vi "UMLEditor PostComment.vi"(1 "name":string="mikael.holmstrom@endevo.se", 3 "comment":string="Hejsan\nHär e mina komments!!\n//Micke", 5 "error in (no error)":errorcluster) -> (19 "error out":errorcluster)   [LabVIEW 2012]
panel:
  out "Text1":string="HTTP/1.0 200 OK\r\nDate: Mon, 28 Apr 2003 08:45:03 GMT\r\nServer: Apache/1.3.20 (Unix) ApacheJServ/1.1.2 PHP/4.2.3 FrontPage/5.0.2.2510 Rewrit/1.1a\r\nContent-Type: text/html\r\nX-Cache: MISS from 217.75.96.62\r\nX-Cache-Lookup: MISS from 217.75.96.62:3128\r\nConnection: close\r\n\r\n<p>Hello, micke!</p>\n<p>holmstrom</p>\n"
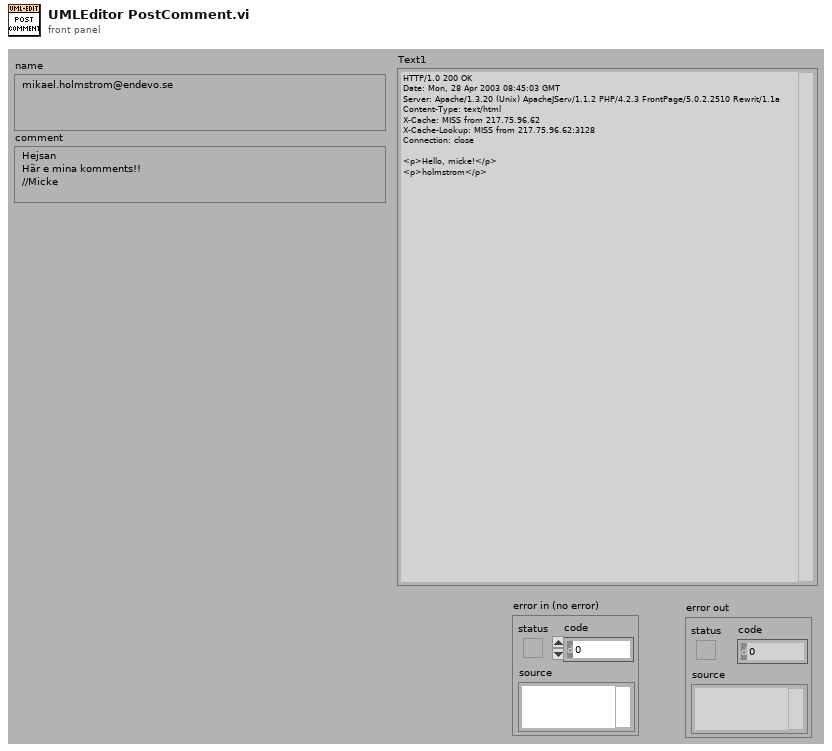
[diagram p1: front panel]
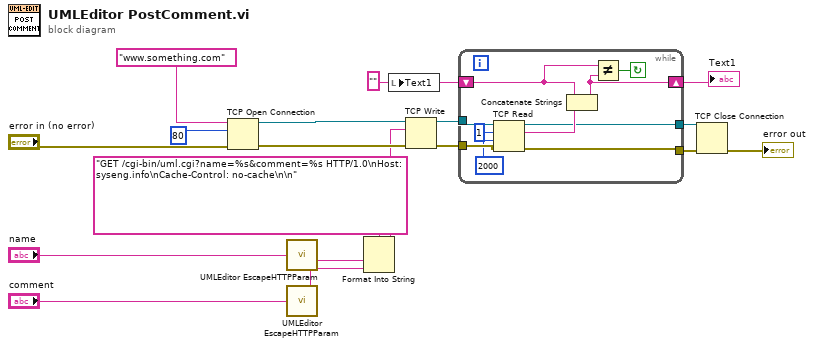
[diagram p0: block diagram]
diagram:
  w18 = "" ("address")
  n1 = TCP Open Connection(address="www.something.com", remote port or service name=u16 80 ("remote port"), error in (no error)="error in (no error)") -> (connection ID=w10:refnum<k5>, error out=w9:errorcluster)  [unwired: 2 out]
  n2 = call <resource>:"UMLEditor EscapeHTTPParam.vi"("string"="name") -> ("url-encoded string"=w6:string)
  n3 = call <resource>:"UMLEditor EscapeHTTPParam.vi"("string"="comment") -> ("url-encoded string"=w5:string)
  n4 = Format Into String(format string="GET /cgi-bin/uml.cgi?name=%s&comment=%s HTTP/1.0\nHost: syseng.info\nCache-Control: no-cache\n\n" ("Text sent"), w6, w5) -> (resulting string=w7:string)  [unwired: 2 in, 1 out]
  n5 = local write "Text1"(w18) -> ()
  n6 = TCP Write(connection ID=w10, data in=w7, error in (no error)=w9) -> (connection ID out=w17:refnum<k5>, error out=w16:errorcluster)  [unwired: 2 out]
  n7 = while {
    tunnel: [w19] -> w14
    tunnel: [w21] -> w15
    tunnel: w16 -> [w22]
    shift-left: w18 -> [w25]
    shift-right: [w24] -> w13
    tunnel: w17 -> [w28]
    stop <- w23 continue-if-true
    n8 = TCP Read(connection ID=w28, bytes to read=1, error in (no error)=w22, 9:2000 ("timeout ms (25000)")) -> (connection ID out=w21:refnum<k5>, data out=w26:string, error out=w19:errorcluster)  [unwired: 1 out]
    n9 = Concatenate Strings(w25, w26) -> (w24:string)
    n10 = Not Equal?(x=w25, y=w24) -> (x != y?=w23:bool)
  }
  "Text1" <- w13
  n11 = TCP Close Connection(connection ID=w15, error in (no error)=w14) -> (error out=→"error out":errorcluster)  [unwired: 2 out]
